vi "Release-framegrabber.vi"(8 "error in":errorcluster, 11 "Data ref. in":refnum<data-value>) -> (0 "error IO":errorcluster, 3 "Data ref.":refnum<data-value>)   [LabVIEW 2013, in "CameraVision.lvlib" / "CV-Main.lvclass"]
uses:
  CV-Main.lvclass
  CV-Main.lvclass/CV-Main.ctl
  Configuration/CV-Configuration.lvclass/CV-Configuration.ctl
  UI/Module-states.ctl
  Read Config params.vi
  Configuration/Read Framegrabber DLL file.vi
  Configuration/Read BoardHandle.vi
  Configuration/Read DMA adresses.vi
  Configuration/Read Camport array.vi
  Configuration/Read Grabber status.vi
  Configuration/CV-Configuration.lvclass
  UI/CV-UI.lvclass
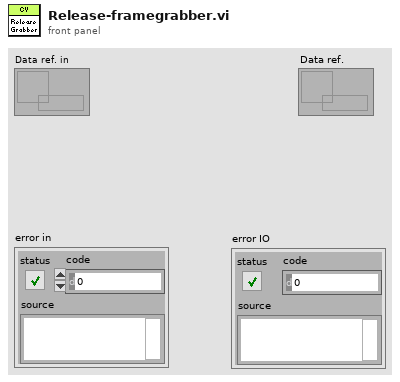
[diagram p1: front panel]
types:
  T1 = typedef "CameraVision.lvlib/CV-UI.lvclass/Module-states.ctl" = enum16{"Inactive", "Active", "Data-loss", "Error", "Simulation", "Synchronizing", "Initialized", "Released"}
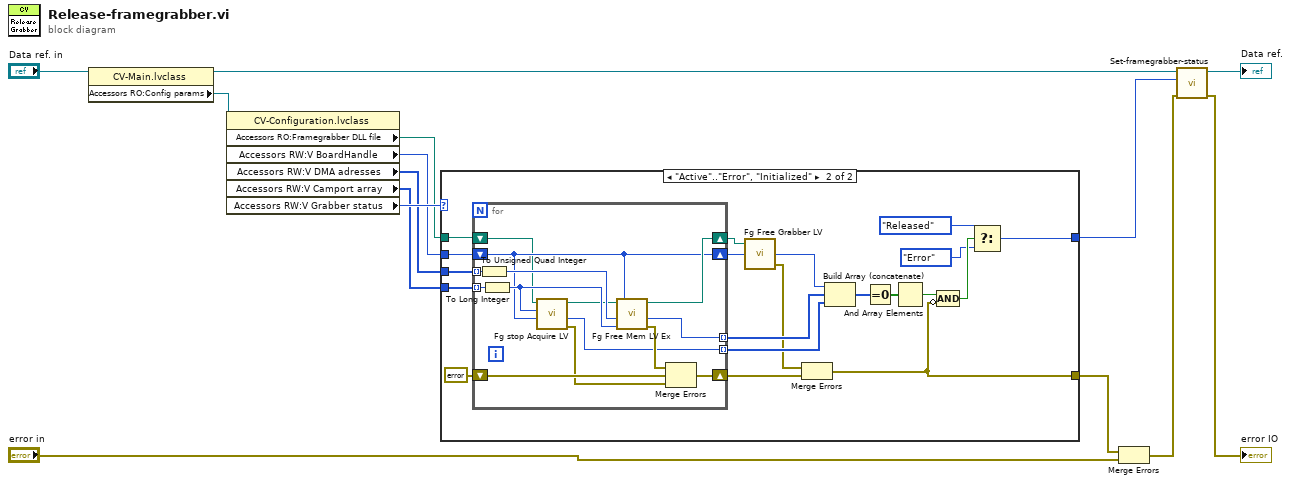
[diagram p0: block diagram]
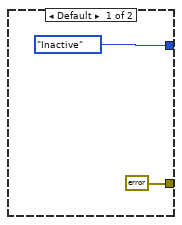
[diagram p2: hidden frame]
diagram:
  n1 = property class="CV-Main.lvclass"(reference="Data ref. in") -> (reference out=w13:refnum<data-value>, "Accessors RO:Config params"=w5:refnum<data-value>)  [unwired: 1 in, 1 out]
  n2 = property class="CV-Configuration.lvclass"(reference=w5) -> ("Accessors RO:Framegrabber DLL file"=w6:path, "Accessors RW:V BoardHandle"=w7:u64, "Accessors RW:V DMA adresses"=w8:i64[], "Accessors RW:V Camport array"=w9:u32[], "Accessors RW:V Grabber status"=w10:T1)  [unwired: 1 in, 2 out]
  n3 = case shown="\"Active\"..\"Error\", \"Initialized\"" w10 {
    tunnel: [errorcluster {"status"=FALSE, "code"=0, "source"=""} ("error IO") w19] -> w11
    tunnel: w9 -> [_ w33]
    tunnel: w7 -> [_ w32]
    tunnel: w6 -> [_ w31]
    tunnel: w8 -> [_ w25]
    tunnel: [Module-states."Inactive" ("Grabber status") w21] -> w1
    frame Default {
    }
    frame "Active".."Error", "Initialized" {
      n4 = for {
        tunnel: w33 -> [w50] mode=indexing
        shift-right: [w46] -> w36
        shift-left: errorcluster {"status"=FALSE, "code"=0, "source"=""} ("error IO") -> [w43]
        shift-right: [w49] -> w30
        shift-left: w31 -> [w38]
        shift-right: [w39] -> w29
        shift-left: w32 -> [w39]
        tunnel: [w48] -> w27 mode=indexing
        tunnel: w25 -> [w45] mode=indexing
        tunnel: [w41] -> w20 mode=indexing
        n5 = To Unsigned Quad Integer(1:w45) -> (0:w44:u64)
        n6 = To Long Integer(number=w50) -> (32bit integer=w40:i32)
        n7 = call <userlib>:"Fg stop Acquire LV.vi"("FgAddr"=w39, "CamPort"=w40, "dll path in"=w38) -> ("error out"=w42:errorcluster, "function return"=w41:i32, "dll path out"=w37:path)  [unwired: 2 in]
        n8 = call <userlib>:"Fg Free Mem LV Ex.vi"("CamPort"=w40, "DMAAddr"=w44, "FgAddr"=w39, "dll path in"=w37) -> ("error out"=w47:errorcluster, "function return"=w48:i32, "dll path out"=w49:path)  [unwired: 1 in]
        n9 = Merge Errors(w47, w43, w42) -> (w46:errorcluster)
      }
      n10 = call <userlib>:"Fg Free Grabber LV.vi"("FgAddr"=w29, "dll path in"=w30) -> ("error out"=w18:errorcluster, "function return"=w28:i32)  [unwired: 1 in, 1 out]
      n11 = Merge Errors(w18, w36) -> (w19:errorcluster)
      n12 = Build Array (concatenate)(w28, w27, w20) -> (w34:i32[])
      n13 = Equal To 0?(x=w34) -> (x = 0?=w35:bool[])
      n14 = And Array Elements(Boolean array=w35) -> (logical AND=w26:bool)
      n15 = Compound Arithmetic op=AND(w26, invert w19) -> (w24:bool)
      n16 = Select(t=Module-states."Released" ("Grabber status"), s=w24, f=Module-states."Error" ("Grabber status")) -> (s? t:f=w21:T1)
    }
  }
  n17 = Merge Errors(w11, "error in") -> (w3:errorcluster)
  n18 = call "Set-framegrabber-status.vi"("error in"=w3, "Grabber status in"=w1, "Data ref. in"=w13) -> ("error IO"=→"error IO":errorcluster, "Data ref."=→"Data ref.":refnum<data-value>)  [unwired: 6 in, 1 out]
